vi "OpenFaultLogger.vi"(8 "Timing Trigger":u16, 9 "Timing Notifier":refnum<notifier>, 10 "BurstSize":u32, 11 "BufferSize":u32) -> (3 "FaultDevRef":T1)   [LabVIEW 2016]
uses:
  Fault_Fifos.ctl
  Faults.ctl
  Fault_Cluster.ctl
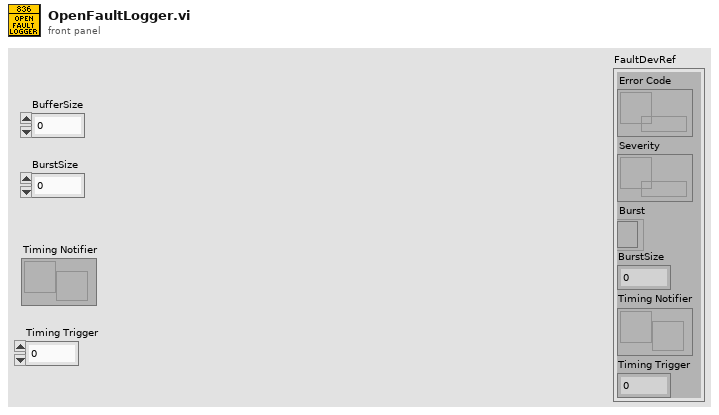
[diagram p1: front panel]
types:
  T1 = typedef "Fault_Fifos.ctl" = cluster{"Error Code":refnum<k33>, "Severity":refnum<k33>, "Burst":refnum<k4>, "BurstSize":u32, "Timing Notifier":refnum<notifier>, "Timing Trigger":u16}
  T2 = typedef "Fault_Cluster.ctl" = cluster{"Error Code":T3, "Severity":u32, "Message":string, "Origin":string}
  T3 = typedef "Faults.ctl" = enum16{"Boiler Target Lost", "Gerar Target Lost", "Body IMU Fault", "Turret IMU Fault"}
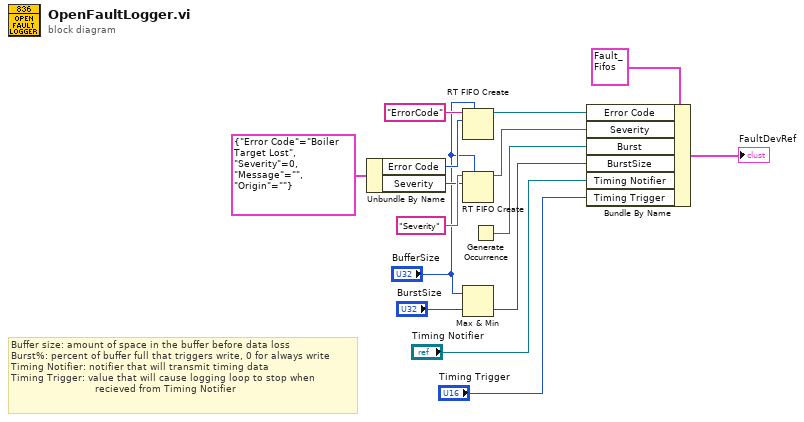
[diagram p0: block diagram]
diagram:
  # "Buffer size: amount of space in the buffer before data loss\nBurst%: percent of buffer full that triggers write, 0 for always write\nTiming Notifier: notifier that will transmit timing data\nTiming Trigger: value that will cause logging loop to stop when\n                            recieved from Timing Notifier"
  n1 = Unbundle By Name(T2 {"Error Code"=enum."Boiler Target Lost", "Severity"=0, "Message"="", "Origin"=""} ("Fault")) -> ("Error Code"=w10:T3, "Severity"=w9:u32)
  n2 = RT FIFO Create(0:"ErrorCode" ("name (unnamed)"), 1:w10, 4:"BufferSize") -> (8:w8:refnum<k33>)  [unwired: 5 in, 2 out]
  n3 = RT FIFO Create(0:"Severity" ("name (unnamed)"), 1:w9, 4:"BufferSize") -> (8:w7:refnum<k33>)  [unwired: 5 in, 2 out]
  n4 = Max & Min(x="BufferSize", y="BurstSize") -> (min(x,y)=w3:u32)  [unwired: 1 out]
  n5 = Generate Occurrence() -> (w6:refnum<k4>)
  n6 = Bundle By Name(cluster=T1 {"Error Code"=refnum, "Severity"=refnum, "Burst"=refnum, "BurstSize"=0, "Timing Notifier"=refnum, "Timing Trigger"=0} ("FaultDevRef"), "Error Code"=w8, "Severity"=w7, "Burst"=w6, "BurstSize"=w3, "Timing Notifier"="Timing Notifier", "Timing Trigger"="Timing Trigger") -> (→"FaultDevRef":T1)
